vi "img_close_file.vi"(8 "error in":errorcluster, 11 "hFile":i64) -> (0 "error out":errorcluster)   [LabVIEW 2016]
uses:
  kernel32.dll
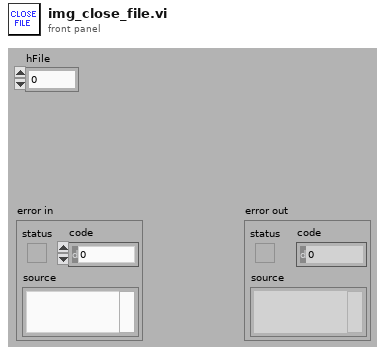
[diagram p1: front panel]
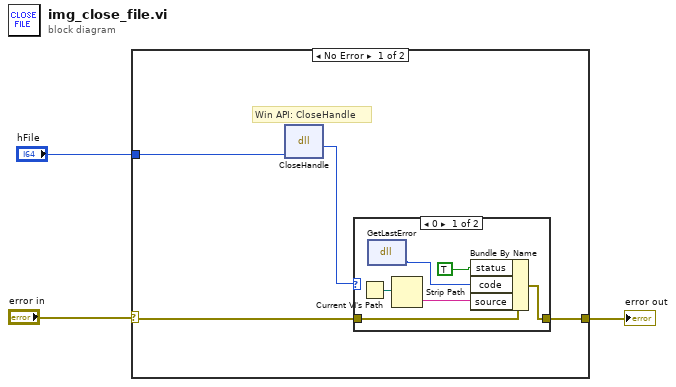
[diagram p0: block diagram]
diagram:
  n1 = case shown="No Error" "error in" {
    selector: "error in" -> [w7 w15]
    tunnel: "hFile" -> [w4 _]
    tunnel: [w6 w15] -> w2
    frame No Error {
      # "Win API: CloseHandle"
      n2 = dll-call lib="kernel32.dll" fn="CloseHandle"("hFile"=w4) -> ("error"=w5:i32)  [unwired: 4 in, 2 out]
      n3 = case shown="0" w5 {
        tunnel: w7 -> [w13 w14]
        tunnel: [w12 w14] -> w6
        frame 0 {
          n4 = Current VI's Path() -> (path=w10:path)
          n5 = dll-call lib="kernel32.dll" fn="GetLastError"() -> ("error"=w8:u32)  [unwired: 3 in, 2 out]
          n6 = Strip Path(path=w10) -> (name=w9:string)  [unwired: 1 out]
          n7 = Bundle By Name(cluster=w13, "status"=TRUE, "code"=w8, "source"=w9) -> (w12:errorcluster)
        }
        frame 1, Default {
        }
      }
    }
    frame Error {
    }
  }
  "error out" <- w2
